vi "Elasped Timer.vi"(8 "error in (no error)":errorcluster, 10 "Time Setting":dbl, 11 "Action":T1) -> (0 "error out":errorcluster, 1 "Elapsed Time":dbl format="%#_2g", 2 "Time Left":dbl format="%#_2g", 3 "Time Out?!":bool)   [LabVIEW 2018]
uses:
  Elapsed timer control.ctl
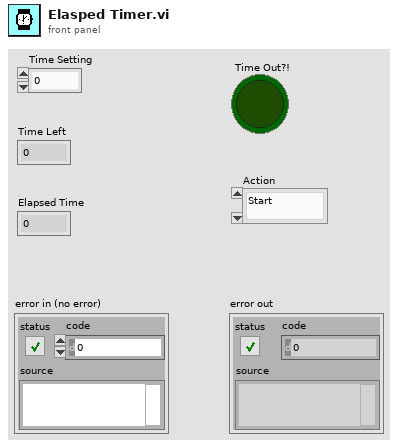
[diagram p1: front panel]
types:
  T1 = typedef "Elapsed timer control.ctl" = enum16{"Start", "Pause", "Initialize"}
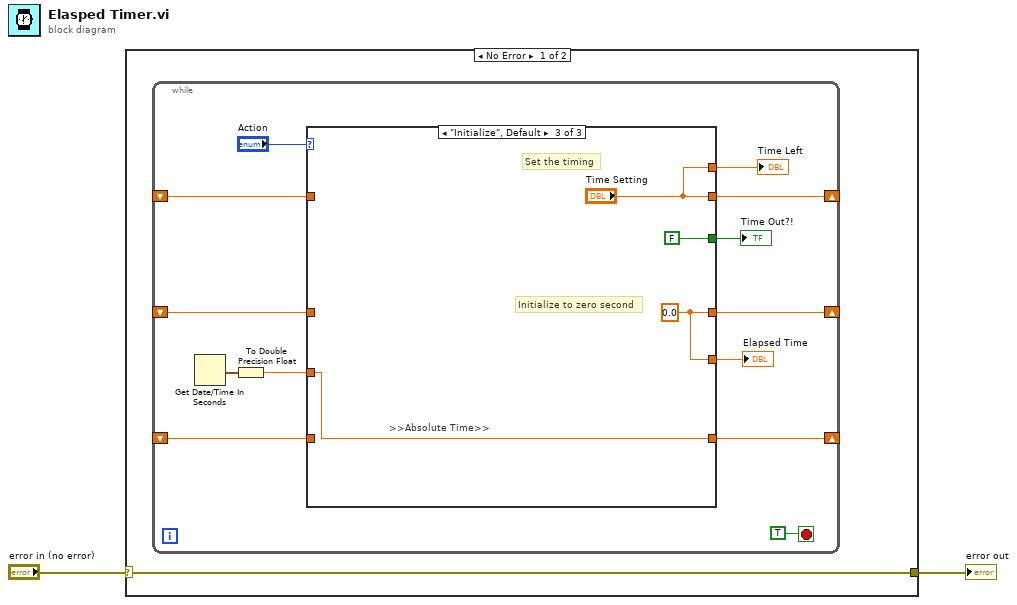
[diagram p0: block diagram]
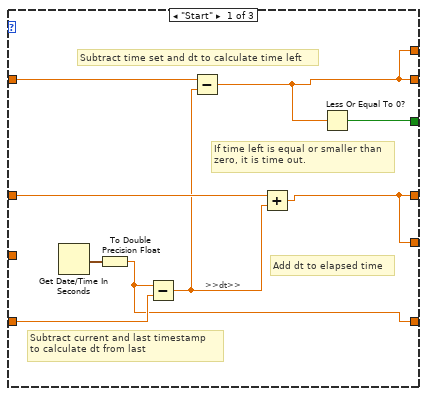
[diagram p2: hidden frame]
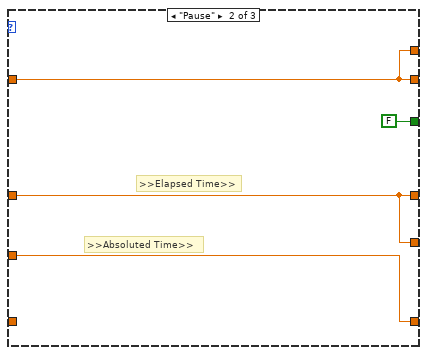
[diagram p3: hidden frame]
diagram:
  n1 = case shown="No Error" "error in (no error)" {
    selector: "error in (no error)" -> [w3 w34]
    tunnel: [w3 w34] -> w1
    frame No Error {
      n2 = while {
        shift-right: [w11] -> _
        shift-left: _ -> [w6]
        shift-right: [w8] -> _
        shift-left: _ -> [w4]
        shift-right: [w13] -> _
        shift-left: _ -> [w5]
        stop <- TRUE stop-if-true
        n3 = Get Date/Time In Seconds() -> (seconds since 1Jan1904=w15:timestamp)
        n4 = To Double Precision Float(number=w15) -> (double precision float=w14:dbl)
        n5 = case shown="\"Initialize\", Default" "Action" {
          tunnel: w14 -> [_ w26 w33]
          tunnel: [w19 w26 w33] -> w13
          tunnel: [w17 w29 "Time Setting"] -> w11
          tunnel: [w17 w29 "Time Setting"] -> w10
          tunnel: [w24 FALSE FALSE] -> w9
          tunnel: [w18 w27 w30] -> w8
          tunnel: [w18 w27 w30] -> w7
          tunnel: w6 -> [w23 w29 _]
          tunnel: w5 -> [w22 _ _]
          tunnel: w4 -> [w21 w27 _]
          frame "Start" {
            # "If time left is equal or smaller than\nzero, it is time out."
            # "Subtract time set and dt to calculate time left"
            # "Add dt to elapsed time"
            # "Subtract current and last timestamp \nto calculate dt from last"
            # ">>dt>>"
            n6 = Get Date/Time In Seconds() -> (seconds since 1Jan1904=w25:timestamp)
            n7 = To Double Precision Float(number=w25) -> (double precision float=w19:dbl)
            n8 = Subtract(x=w19, y=w22) -> (x-y=w20:dbl)
            n9 = Subtract(x=w23, y=w20) -> (x-y=w17:dbl)
            n10 = Add(x=w21, y=w20) -> (x+y=w18:dbl)
            n11 = Less Or Equal To 0?(x=w17) -> (x <= 0?=w24:bool)
          }
          frame "Pause" {
            # ">>Elapsed Time>>"
            # ">>Absoluted Time>>"
          }
          frame "Initialize", Default {
            w30 = 0.0
            # ">>Absolute Time>>"
            # "Set the timing"
            # "Initialize to zero second"
          }
        }
        "Time Left" <- w10
        "Elapsed Time" <- w7
        "Time Out?!" <- w9
      }
    }
    frame Error {
    }
  }
  "error out" <- w1
